vi "시간.vi"() -> ()   [LabVIEW 2014]
panel:
  out "초단위":dbl
  in  "시간입력":dbl
  in  "링":u32(ring) items=["초"=1, "분"=60, "시간"=3600, "하루"=86400]
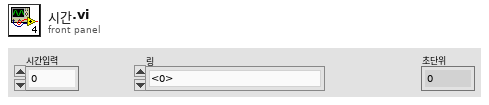
[diagram p1: front panel]
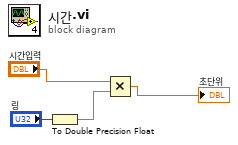
[diagram p0: block diagram]
diagram:
  n1 = To Double Precision Float(number="링") -> (double precision float=w1:dbl)
  n2 = Multiply(x="시간입력", y=w1) -> (x*y=→"초단위":dbl)
